vi "Example 3 trig in_out.vi"() -> ()   [LabVIEW 2015]
uses:
  <vilib>/Platform/TimedLoop/XDataNode/timing_clust.ctl
  <vilib>/Platform/TimedLoop/XDataNode/nitl_modes.ctl
  <vilib>/Platform/TimedLoop/XDataNode/wakeup.ctl
  <vilib>/Platform/TimedLoop/XDataNode/XDataNode.xnode
  <vilib>/Platform/TimedLoop/XDataNode/XDNodeRunTimeDep.lvlib
panel:
  out "read 7":dbl
  out "read 6":dbl
  in  "Trigger Out Mode S":u16(ring)=2 items=["OFF", "TRIG", "FSTR"]
  in  "Trigger Out Mode M":u16(ring)=2 items=["OFF", "TRIG", "FSTR"]
  out "resulting string":string="loop -1 from 1"
  out "Counter":dbl=1.0
  in  "Trigger in Delay M(s)":dbl=1.0
  out "full master program time[s]":dbl=4.0
  in  "stop":bool
  in  "Language Selector":i16(ring)=1 items=["GEN", "SCPI"]
  in  "Baud Rate":i32(ring)=6 items=["1200", "2400", "4800", "9600", "19200", "38400", "57600", "115200"]
  in  "Address":i16=6
  out "Read Set Voltage":dbl=5.0
  in  "dt":dbl=0.02 step=0.001 format="%#4_6g"
  in  "time screen\n [SEC]":i16(knob)=10 scale=0.0..60.0
  in  "Trigger in Delay S(s)":dbl=1.0
  out "Waveform Graph":dynamicdata(graph)=[{"t0"=timestamp(0 s since 1904-01-01), "dt"=0.02, "Y"=[-1.0, -1.0, -1.0, -1.0, -1.0, -1.0, -1.0, -1.0, -1.0, -1.0, -1.0, -1.0, -1.0, -1.0, -1.0, -1.0, -1.0, -1.0, -1.0, -1.0, -1.0, -1.0, -1.0, -1.0, -1.0, -1.0, -1.0, -1.0, -1.0, -1.0, -1.0, -1.0, -1.0, -1.0, -1.0, -1.0, -1.0, -1.0, -1.0, -1.0, -1.0, -1.0, -1.0, -1.0, -1.0, -1.0, -1.0, -1.0, -1.0, -1.0, -1.0, -1.0, -1.0, -1.0, -1.0, -1.0, -1.0, -1.0, -1.0, -1.0, -1.0, -1.0, -1.0, -1.0, -1.0, -1.0, -1.0, -1.0, -1.0, -1.0, -1.0, -1.0, -1.0, -1.0, -1.0, -1.0, -1.0, -1.0, -1.0, -1.0, -1.0, -1.0, -1.0, -1.0, -1.0, -1.0, -1.0, -1.0, -1.0, -1.0, -1.0, -1.0, -1.0, -1.0, -1.0, -1.0, -1.0, -1.0, -1.0, -1.0, -1.0, -1.0, -1.0, -1.0, -1.0, -1.0, -1.0, -1.0, -1.0, -1.0, -1.0, -1.0, -1.0, -1.0, -1.0, -1.0, -1.0, -1.0, -1.0, -1.0, -1.0, -1.0, -1.0, -1.0, -1.0, -1.0, -1.0, -1.0, -1.0, -1.0, -1.0, -1.0, -1.0, -1.0, -1.0, -1.0, -1.0, -1.0, -1.0, -1.0, -1.0, -1.0, -1.0, -1.0, -1.0, -1.0, -1.0, -1.0, -1.0, -1.0, -1.0, -1.0, -1.0, -1.0, -1.0, -1.0, -1.0, -1.0, -1.0, -1.0, -1.0, -1.0, -1.0, -1.0, -1.0, -1.0, -1.0, -1.0, -1.0, -1.0, -1.0, -1.0, -1.0, -1.0, -1.0, -1.0, -1.0, -1.0, -1.0, -1.0, -1.0, -1.0, -1.0, -1.0, -1.0, -1.0, -1.0, -1.0, -1.0, -1.0, -1.0, -1.0, -1.0, -1.0, -1.0, -1.0, -1.0, -1.0, -1.0, -1.0, -1.0, -1.0, -1.0, -1.0, -1.0, -1.0, -1.0, -1.0, -1.0, -1.0, -1.0, -1.0, -1.0, -1.0, -1.0, -1.0, -1.0, -1.0, -1.0, -1.0, -1.0, -1.0, -1.0, -1.0, -1.0, -1.0, -1.0, -1.0, -1.0, -1.0, -1.0, -1.0, -1.0, -1.0, -1.0, -1.0, -1.0, -1.0, -1.0, -1.0, -1.0, -1.0, -1.0, -1.0, -1.0, -1.0, -1.0, -1.0, -1.0, -1.0, -1.0, -1.0, -1.0, -1.0, -1.0, -1.0, -1.0, -1.0, -1.0, -1.0, -1.0, -1.0, -1.0, -1.0, -1.0, -1.0, -1.0, -1.0, -1.0, -1.0, -1.0, -1.0, -1.0, -1.0, -1.0, -1.0, -1.0, -1.0, -1.0, -1.0, -1.0, -1.0, -1.0, -1.0, -1.0, -1.0, -1.0, -1.0, -1.0, -1.0, -1.0, -1.0, -1.0, -1.0, -1.0, -1.0, -1.0, -1.0, -1.0, -1.0, -1.0, -1.0, -1.0, -1.0, -1.0, -1.0, -1.0, -1.0, -1.0, -1.0, -1.0, -1.0, -1.0, -1.0, -1.0, -1.0, -1.0, -1.0, -1.0, -1.0, -1.0, -1.0, -1.0, -1.0, -1.0, -1.0, -1.0, -1.0, -1.0, -1.0, -1.0, -1.0, -1.0, -1.0, -1.0, -1.0, -1.0, -1.0, -1.0, -1.0, -1.0, -1.0, -1.0, -1.0, -1.0, -1.0, -1.0, -1.0, -1.0, -1.0, -1.0, -1.0, -1.0, -1.0, -1.0, -1.0, -1.0, -1.0, -1.0, -1.0, -1.0, -1.0, -1.0, -1.0, -1.0, -1.0, -1.0, -1.0, -1.0, -1.0, -1.0, -1.0, -1.0, -1.0, -1.0, -1.0, -1.0, -1.0, -1.0, -1.0, -1.0, -1.0, -1.0, -1.0, -1.0, -1.0, -1.0, -1.0, -1.0, -1.0, -1.0, -1.0, -1.0, -1.0, -1.0, -1.0, -1.0, -1.0, -1.0, -1.0, -1.0, -1.0, -1.0, -1.0, -1.0, -1.0, -1.0, -1.0, -1.0, -1.0, -1.0, -1.0, -1.0, -1.0, -1.0, -1.0, -1.0, -1.0, -1.0, -1.0, -1.0, -1.0, -1.0, -1.0, -1.0, -1.0, -1.0, -1.0, -1.0, -1.0, -1.0, -1.0, -1.0, -1.0, -1.0, -1.0, -1.0, -1.0, -1.0, -1.0, -1.0, -1.0, -1.0, -1.0, -1.0, -1.0, -1.0, -1.0, -1.0, -1.0, -1.0, -1.0, -1.0, -1.0, -1.0, -1.0, -1.0, -1.0, -1.0, -1.0, -1.0, -1.0, -1.0, -1.0, -1.0, -1.0, -1.0, -1.0, -1.0, -1.0, -1.0, -1.0, -1.0, -1.0, -1.0, -1.0, -1.0, -1.0, -1.0, -1.0, -1.0, -1.0, -1.0, -1.0, -1.0, -1.0, -1.0, -1.0, -1.0, -1.0, -1.0, -1.0, -1.0, -1.0, -1.0, -1.0, -1.0, -1.0, -1.0, -1.0]}, {"t0"=timestamp(0 s since 1904-01-01), "dt"=0.02, "Y"=[0.0, 0.0, 0.0, 0.0, 0.0, 0.0, 0.0, 0.0, 0.0, 0.0, 0.0, 0.0, 0.0, 0.0, 0.0, 0.0, 0.0, 0.0, 0.0, 0.0, 0.0, 0.0, 0.0, 0.0, 0.0, 0.0, 0.0, 0.0, 0.0, 0.0, 0.0, 0.0, 0.0, 0.0, 0.0, 0.0, 0.0, 0.0, 0.0, 0.0, 0.0, 0.0, 0.0, 0.0, 0.0, 0.0, 0.0, 0.0, 0.0, 0.0, 0.0, 0.0, 0.0, 0.0, 0.0, 0.0, 0.0, 0.0, 0.0, 0.0, 0.0, 0.0, 0.0, 0.0, 0.0, 0.0, 0.0, 0.0, 0.0, 0.809, 0.809, 1.598, 1.598, 2.408, 2.408, 3.207, 3.207, 4.006, 4.006, 4.805, 4.805, 5.594, 5.594, 6.394, 6.394, 7.203, 7.203, 8.002, 8.002, 8.801, 8.801, 9.6, 9.6, 10.0, 10.0, 10.0, 10.0, 10.0, 10.0, 10.0, 10.0, 10.0, 10.0, 10.0, 10.0, 10.0, 10.0, 10.0, 10.0, 10.0, 10.0, 10.0, 10.0, 10.0, 10.0, 10.0, 10.0, 10.0, 10.0, 10.0, 10.0, 10.0, 10.0, 10.0, 10.0, 10.0, 10.0, 10.0, 10.0, 10.0, 10.0, 10.0, 10.0, 10.0, 10.0, 10.0, 10.0, 10.0, 10.0, 10.0, 10.0, 10.0, 10.0, 9.84, 9.84, 9.52, 9.52, 9.197, 9.197, 8.877, 8.877, 8.557, 8.557, 8.246, 8.246, 7.926, 7.926, 7.602, 7.602, 7.279, 7.279, 6.959, 6.959, 6.639, 6.639, 6.324, 6.324, 6.004, 6.004, 6.0, 6.0, 6.0, 6.0, 6.0, 6.0, 6.0, 6.0, 6.0, 6.0, 6.0, 6.0, 6.0, 6.0, 6.0, 6.0, 6.0, 6.0, 6.0, 6.0, 6.0, 6.0, 6.0, 6.0, 6.0, 6.0, 6.0, 6.0, 6.0, 6.0, 6.0, 6.0, 6.0, 6.0, 6.0, 6.0, 6.0, 6.0, 6.0, 6.0, 6.0, 6.0, 6.0, 6.0, 6.0, 6.0, 6.0, 6.0, 6.0, 6.0, 6.162, 6.162, 6.319, 6.319, 6.481, 6.481, 6.641, 6.641, 6.803, 6.803, 6.957, 6.957, 7.119, 7.119, 7.28, 7.28, 7.44, 7.44, 7.6, 7.6, 7.76, 7.76, 7.922, 7.922, 8.0, 8.0, 8.0, 8.0, 8.0, 8.0, 8.0, 8.0, 8.0, 8.0, 8.0, 8.0, 8.0, 8.0, 8.0, 8.0, 8.0, 8.0, 8.0, 8.0, 8.0, 8.0, 8.0, 8.0, 8.0, 8.0, 8.0, 8.0, 8.0, 8.0, 8.0, 8.0, 8.0, 8.0, 8.0, 8.0, 8.0, 8.0, 8.0, 8.0, 8.0, 8.0, 8.0, 8.0, 8.0, 8.0, 8.0, 8.0]}, {"t0"=timestamp(0 s since 1904-01-01), "dt"=0.02, "Y"=[0.0, 0.0, 0.0, 0.0, 0.0, 0.0, 0.0, 0.0, 0.0, 0.0, 0.0, 0.0, 0.0, 0.0, 0.0, 0.0, 0.0, 0.0, 0.195, 0.195, 0.594, 0.594, 0.999, 0.999, 1.399, 1.399, 1.798, 1.798, 2.203, 2.203, 2.597, 2.597, 2.992, 2.992, 3.396, 3.396, 3.796, 3.796, 4.191, 4.191, 4.59, 4.59, 4.99, 4.99, 5.0, 5.0, 5.0, 5.0, 5.0, 5.0, 5.0, 5.0, 5.0, 5.0, 5.0, 5.0, 5.0, 5.0, 5.0, 5.0, 5.0, 5.0, 5.0, 5.0, 5.0, 5.0, 5.0, 5.0, 5.0, 5.0, 5.0, 5.0, 5.0, 5.0, 5.0, 5.0, 5.0, 5.0, 5.0, 5.0, 5.0, 5.0, 5.0, 5.0, 5.0, 5.0, 5.0, 5.0, 5.0, 5.0, 5.0, 5.0, 5.0, 5.0, 4.84, 4.84, 4.68, 4.68, 4.518, 4.518, 4.358, 4.358, 4.198, 4.198, 4.041, 4.041, 3.881, 3.881, 3.719, 3.719, 3.559, 3.559, 3.399, 3.399, 3.241, 3.241, 3.08, 3.08, 3.0, 3.0, 3.0, 3.0, 3.0, 3.0, 3.0, 3.0, 3.0, 3.0, 3.0, 3.0, 3.0, 3.0, 3.0, 3.0, 3.0, 3.0, 3.0, 3.0, 3.0, 3.0, 3.0, 3.0, 3.0, 3.0, 3.0, 3.0, 3.0, 3.0, 3.0, 3.0, 3.0, 3.0, 3.0, 3.0, 3.0, 3.0, 3.0, 3.0, 3.0, 3.0, 3.0, 3.0, 3.0, 3.0, 3.0, 3.0, 3.0, 3.0, 3.04, 3.04, 3.12, 3.12, 3.201, 3.201, 3.28, 3.28, 3.36, 3.36, 3.438, 3.438, 3.519, 3.519, 3.6, 3.6, 3.68, 3.68, 3.76, 3.76, 3.84, 3.84, 3.92, 3.92, 3.999, 3.999, 4.0, 4.0, 4.0, 4.0, 4.0, 4.0, 4.0, 4.0, 4.0, 4.0, 4.0, 4.0, 4.0, 4.0, 4.0, 4.0, 4.0, 4.0, 4.0, 4.0, 4.0, 4.0, 4.0, 4.0, 4.0, 4.0, 4.0, 4.0, 4.0, 4.0, 4.0, 4.0, 4.0, 4.0, 4.0, 4.0, 4.0, 4.0, 4.0, 4.0, 4.0, 4.0, 4.0, 4.0, 4.0, 4.0, 4.0, 4.0, 4.0, 4.0, 4.079, 4.079, 4.159, 4.159, 4.24, 4.24, 4.321, 4.321, 4.401, 4.401, 4.479, 4.479, 4.559, 4.559, 4.64, 4.64, 4.72, 4.72, 4.8, 4.8, 4.88, 4.88, 4.961, 4.961, 5.0, 5.0, 5.0, 5.0, 5.0, 5.0, 5.0, 5.0, 5.0, 5.0, 5.0, 5.0, 5.0, 5.0, 5.0, 5.0, 5.0, 5.0, 5.0, 5.0, 5.0, 5.0, 5.0]}]
  in  "Boolean":bool
  in  "S DATA":T1={"Value string"="10,6,8", "Time string"="1,1,1", "step"=0, "Counter"=1.0} {"Counter" min=1.0 max=65534.0 step=1.0; "step" items=["ONCE", "AUTO"]}
  in  "S MODE":T2={"Progr Mode"=3, "Mode"=0, "init:cont"=1} {"init:cont" items=["0", "1"]; "Mode" items=["VOLTAGE", "CURRENT"]; "Progr Mode" items=["NONE", "FIX", "LIST", "WAVE"]}
  in  "M DATA":T1={"Value string"="5,3,4", "Time string"="1,1,1", "step"=0, "Counter"=1.0} {"Counter" min=1.0 max=65534.0 step=1.0; "step" items=["ONCE", "AUTO"]}
  in  "M MODE":T2={"Progr Mode"=3, "Mode"=0, "init:cont"=1} {"init:cont" items=["0", "1"]; "Mode" items=["VOLTAGE", "CURRENT"]; "Progr Mode" items=["NONE", "FIX", "LIST", "WAVE"]}
  in  "VISA":refnum<visa-resource-name>="COM10"
  # "Application for two power supplies connected\ndaisy chain with Tr_IN and TR_Out"
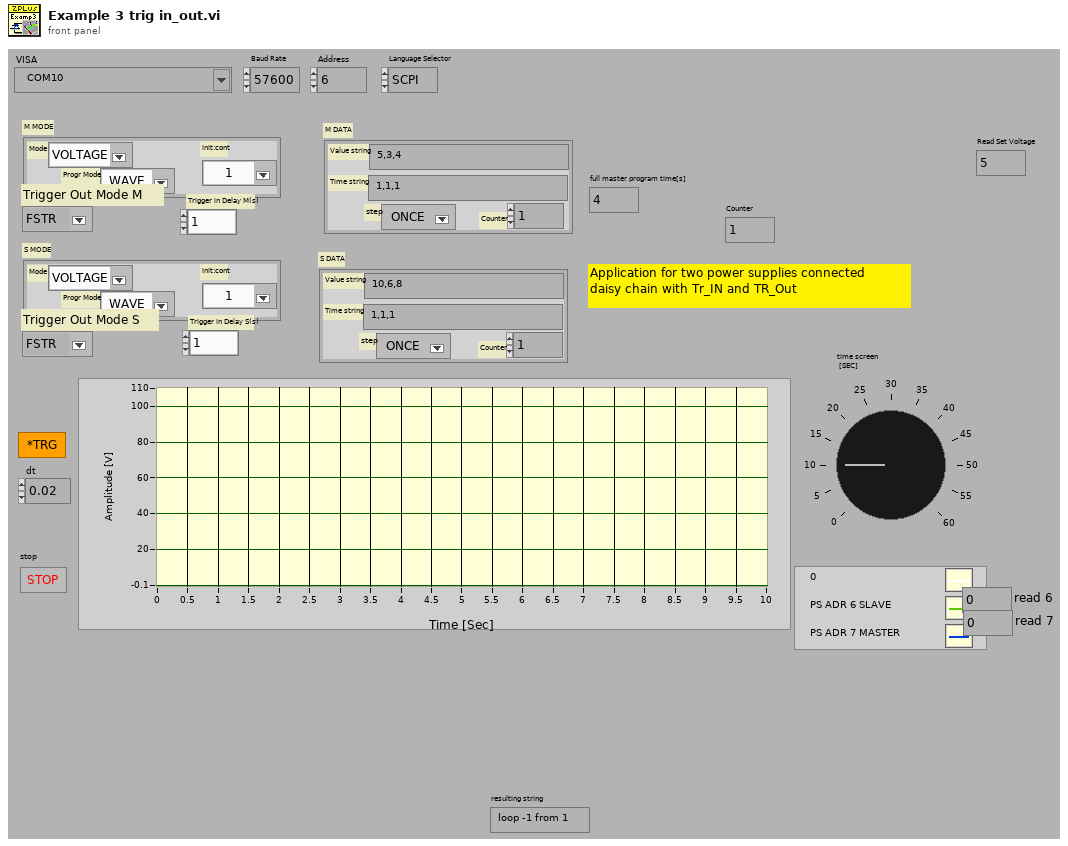
[diagram p1: front panel]
types:
  T1 = cluster{"Value string":string, "Time string":string, "step":u16, "Counter":dbl}
  T2 = cluster{"Progr Mode":u16, "Mode":u16, "init:cont":u16}
  T3 = typedef "XDNodeRunTimeDep.lvlib/timing_clust.ctl" = cluster{"Expected End [f-1]":u64, "Actual End [f-1]":u64, "Finished Late? [f-1]":bool, "Expected End [i-1]":u64, "Actual End [i-1]":u64, "Finished Late? [i-1]":bool, "Expected Start [i]":u64, "Actual Start [i]":u64, "Expected Start [f]":u64, "Actual Start [f]":u64, "Source Name":string, "Structure Name":string, "Period":i64, "Deadline":i64, "Offset":i64, "Start":i64, "Priority":i32, "Timeout":i32, "Mode":T4, "Wakeup Reason":T5, "Error":errorcluster, "Source Type":string, "Secondary Source Type":string, "Global End Time":u64, "Global Start Time":u64, "Frame Duration":u64, "Iteration Duration":u64, "Assigned CPU":i32, "I/O Scan Engine Mode":u32}
  T4 = typedef "XDNodeRunTimeDep.lvlib/nitl_modes.ctl" = enum32{"No Change", "Process missed periods, maintain original phase", "Discard missed periods, maintain original phase", "Process missed periods, ignore original phase", "Discard missed periods, ignore original phase"}
  T5 = typedef "XDNodeRunTimeDep.lvlib/wakeup.ctl" = enum32{"Normal", "Aborted", "Asynchronous wakeup", "Timing source error", "Timed loop error", "Timeout"}
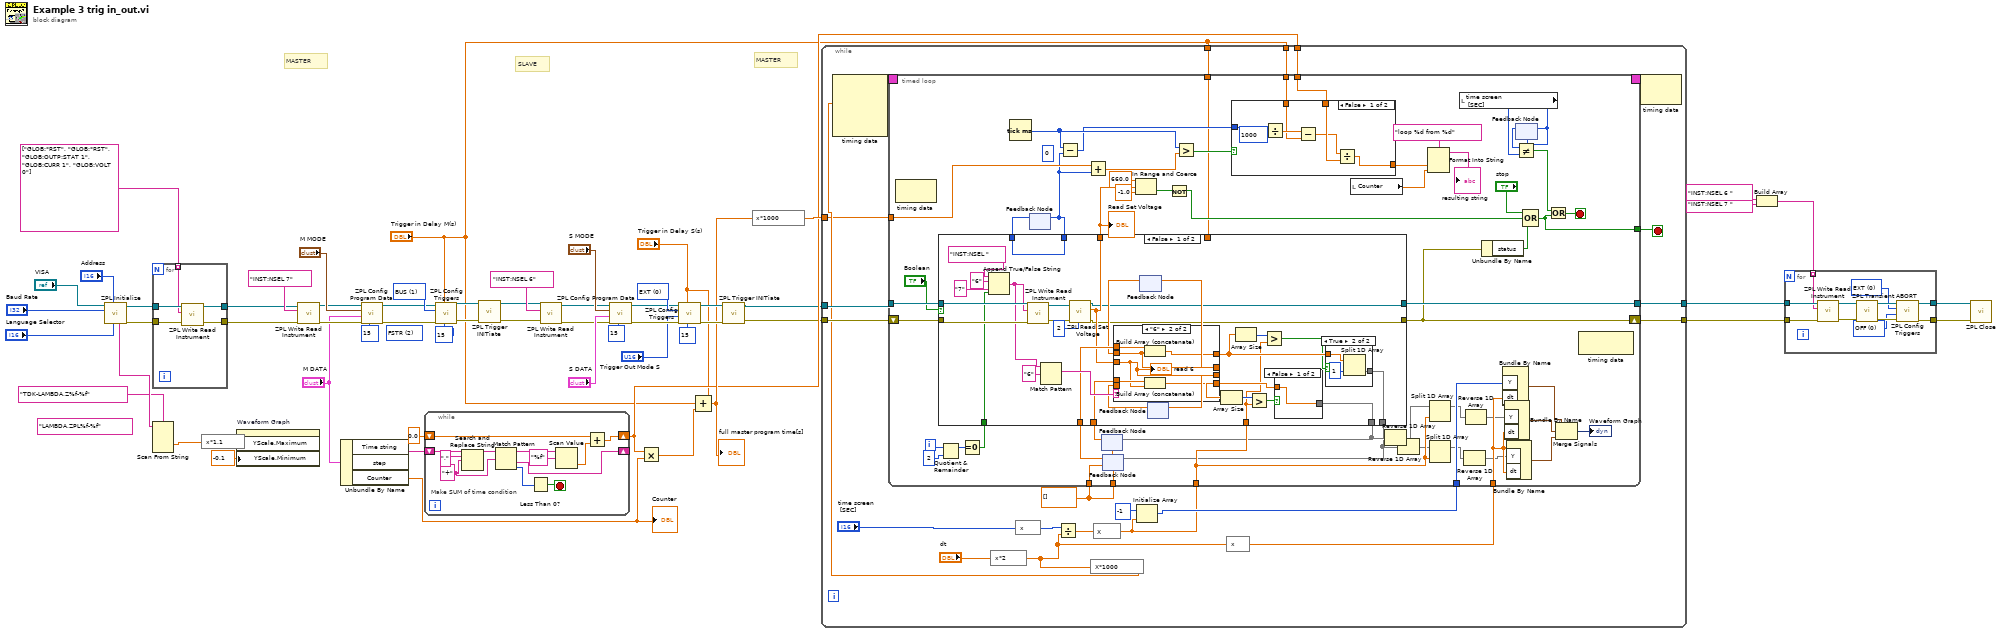
[diagram p0: block diagram]
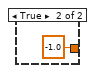
[diagram p2: hidden frame]
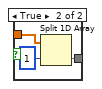
[diagram p4: hidden frame]
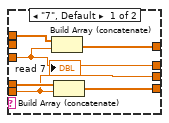
[diagram p5: hidden frame]
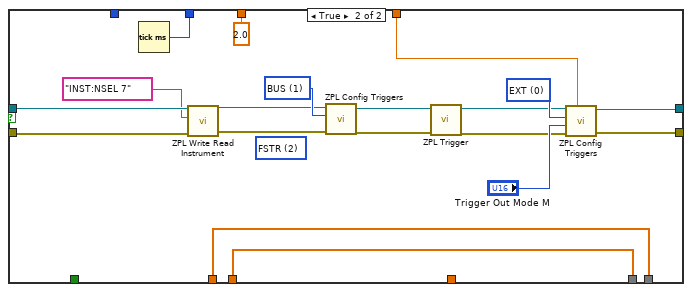
[diagram p6: hidden frame]
diagram:
  (unwired) "LAMBDA,ZPL%f-%f" ("format string")
  (unwired) u16 2 items=["OFF", "TRIG", "FSTR"] ("Trigger Out Mode")
  w50 = u16 0 items=["EXT", "BUS"] ("Trigger in  Source")
  w54 = u16 1 items=["EXT", "BUS"] ("Trigger in  Source")
  # "MASTER"
  # "SLAVE"
  # "MASTER"
  n1 = call "ZPL Initialize.vi"("Language Selector"="Language Selector", "Address"="Address", "Baud Rate"="Baud Rate", "VISA"="VISA") -> ("error out"=w34:errorcluster, "VISA  out"=w33:refnum<visa-resource-name>, "ID responce"=w25:string)  [unwired: 4 in, 1 out]
  n2 = Scan From String(format string="TDK-LAMBDA,Z%f-%f", input string=w25) -> (output 1=w24:dbl)  [unwired: 5 in, 3 out]
  n3 = for {
    tunnel: w34 -> [w64]
    tunnel: w33 -> [w63]
    tunnel: [w62] -> w32
    tunnel: [w61] -> w31
    tunnel: string[] ["GLOB:*RST", "GLOB:*RST", "GLOB:OUTP:STAT 1", "GLOB:CURR 1", "GLOB:VOLT 0"] -> [w60] mode=indexing
    n4 = call "ZPL Write Read Instrument.vi"("error in"=w64, "Write Command/Query SCPI"=w60, "VISA"=w63) -> ("error out"=w61:errorcluster, "VISA  out"=w62:refnum<visa-resource-name>)  [unwired: 6 in, 1 out]
  }
  n5 = expression code="x*1.1"(w24) -> (w23:dbl)
  n6 = property on="Waveform Graph" class="WFGraph (strict)"("YScale.Maximum"=w23, "YScale.Minimum"=-0.1 ("Y Scale.Range:Minimum")) -> ()  [unwired: 2 in, 2 out]
  n7 = call "ZPL Write Read Instrument.vi"("error in"=w31, "Write Command/Query SCPI"="INST:NSEL 7", "VISA"=w32) -> ("error out"=w29:errorcluster, "VISA  out"=w30:refnum<visa-resource-name>)  [unwired: 6 in, 1 out]
  n8 = Unbundle By Name("M DATA") -> ("Time string"=w20:string, "Counter"=w15:dbl)  [unwired: 1 out]
  "Counter" <- w15
  n9 = call "ZPL Config Program Data.vi"("Settle (1 mS)"=u32 15, "error"=w29, "DATA"="M DATA", "MODE"="M MODE", "VISA"=w30) -> ("error out"=w52:errorcluster, "VISA out"=w53:refnum<visa-resource-name>)  [unwired: 4 in, 1 out]
  n10 = while {
    shift-right: [w74] -> _
    shift-left: w20 -> [w73]
    shift-right: [w67] -> w14
    shift-left: 0.0 -> [w66]
    stop <- w71 stop-if-true
    w65 = "+" ("search string")
    # "Make SUM of time condition"
    n11 = Search and Replace String(input string=w73, search string=",", replace string=w65) -> (result string=w75:string)  [unwired: 5 in, 3 out]
    n12 = Match Pattern(string=w75, regular expression=w65) -> (before substring=w69:string, after substring=w74:string, offset past match=w72:i32)  [unwired: 1 in, 1 out]
    n13 = Less Than 0?(x=w72) -> (x < 0?=w71:bool)
    n14 = Scan Value(string=w69, format string="%f") -> (value=w68:dbl)  [unwired: 1 in, 1 out]
    n15 = Add(x=w66, y=w68) -> (x+y=w67:dbl)
  }
  n16 = call "ZPL Config Triggers.vi"("Settle (1 mS)"=u32 15, "Trigger in Delay"="Trigger in Delay M(s)", "error"=w52, "Trigger in  Source"=w54, "VISA"=w53) -> ("error out"=w43:errorcluster, "VISA out"=w44:refnum<visa-resource-name>)  [unwired: 4 in, 1 out]
  n17 = call "ZPL Trigger INITiate.vi"("error"=w43, "VISA"=w44) -> ("error out"=w38:errorcluster, "VISA out"=w42:refnum<visa-resource-name>)  [unwired: 8 in]
  n18 = call "ZPL Write Read Instrument.vi"("error in"=w38, "Write Command/Query SCPI"="INST:NSEL 6", "VISA"=w42) -> ("error out"=w27:errorcluster, "VISA  out"=w28:refnum<visa-resource-name>)  [unwired: 6 in, 1 out]
  n19 = call "ZPL Config Program Data.vi"("Settle (1 mS)"=u32 15, "error"=w27, "DATA"="S DATA", "MODE"="S MODE", "VISA"=w28) -> ("error out"=w48:errorcluster, "VISA out"=w49:refnum<visa-resource-name>)  [unwired: 4 in, 1 out]
  n20 = Multiply(x=w14, y=w15) -> (x*y=w18:dbl)
  n21 = call "ZPL Config Triggers.vi"("Settle (1 mS)"=u32 15, "Trigger in Delay"="Trigger in Delay S(s)", "error"=w48, "Trigger Out Mode"="Trigger Out Mode S", "Trigger in  Source"=w50, "VISA"=w49) -> ("error out"=w40:errorcluster, "VISA out"=w41:refnum<visa-resource-name>)  [unwired: 3 in, 1 out]
  n22 = Compound Arithmetic op=ADD("Trigger in Delay S(s)", "Trigger in Delay M(s)", w18) -> (w17:dbl)
  "full master program time[s]" <- w17
  n23 = call "ZPL Trigger INITiate.vi"("error"=w40, "VISA"=w41) -> ("error out"=w3:errorcluster, "VISA out"=w4:refnum<visa-resource-name>)  [unwired: 8 in]
  n24 = expression code="x*1000"(w17) -> (w19:dbl)
  n25 = while {
    tunnel: [w96] -> w11
    tunnel: [w95] -> w12
    tunnel: w4 -> [w94]
    tunnel: w3 -> [w93]
    tunnel: w19 -> [w81]
    tunnel: w14 -> [w80]
    tunnel: "Trigger in Delay M(s)" -> [w79]
    tunnel: "Trigger in Delay M(s)" -> [w77]
    stop <- w82 stop-if-true
    w91 = dbl[] []
    n26 = expression code="x*2"("dt") -> (w78:dbl)
    n27 = expression code="x"("time screen\n [SEC]") -> (w83:i16)
    n28 = Divide(x=w83, y=w78) -> (x/y=w89:dbl)
    n29 = expression code="X*1000"(w78) -> (w87:dbl)
    n30 = node-c288(w87) -> (w98:T3)  [unwired: 3 in]
    n31 = expression code="X"(w89) -> (w86:dbl)
    n32 = Initialize Array(-1 ("Read Set Voltage"), w86) -> (w90:i32[])
    n33 = expression code="x"(w78) -> (w85:dbl)
    n34 = timed-loop {
      tunnel: w94 -> [w152]
      tunnel: [w136] -> w96
      tunnel: w91 -> [w140]
      tunnel: w91 -> [w139]
      tunnel: w90 -> [w138]
      tunnel: w85 -> [w137]
      tunnel: w86 -> [w108]
      timing: w98 -> [_]
      timing-out: [_] -> w97
      shift-right: [w135] -> w95
      shift-left: w93 -> [w151]
      tunnel: [w125] -> w82
      tunnel: w81 -> [w120]
      tunnel: w80 -> [w114]
      tunnel: w79 -> [w113]
      tunnel: w77 -> [w99]
      i -> [w149]
      stop <- w126 stop-if-true
      (unwired) u32 0 ("y")
      n35 = node-c288() -> ()  [unwired: 1 in, 1 out]
      n36 = Quotient & Remainder(x=w149, y=2) -> (x-y*floor(x/y)=w147:i32)  [unwired: 1 out]
      n37 = Equal To 0?(x=w147) -> (x = 0?=w146:bool)
      n38 = Tick Count (ms)() -> (millisecond timer value=w118:u32)
      n39 = feedback #1() -> (w121:u32)  [unwired: 1 in]
      n40 = feedback #2(w139) -> (w145:dbl[])
      n41 = feedback #3(w140) -> (w144:dbl[])
      n42 = case shown="False" "Boolean" {
        tunnel: w152 -> [w193 w217]
        tunnel: w151 -> [w192 w216]
        tunnel: [w165 w223] -> w136
        tunnel: [w164 w222] -> w135
        tunnel: w146 -> [w189 _]
        tunnel: [w178 w232] -> w107
        tunnel: w145 -> [w182 w232]
        tunnel: [w176 w231] -> w106
        tunnel: w144 -> [w181 w231]
        tunnel: w108 -> [w172 _]
        tunnel: [w167 2.0 ("Read Set Voltage")] -> w133
        tunnel: [w166 w229] -> w117
        tunnel: w121 -> [w166 _]
        tunnel: w99 -> [_ w214]
        frame False {
          n43 = Append True/False String(1:w189, 2:"7" ("false string"), 3:"6" ("true string"), 4:"INST:NSEL " ("Write Command/Query SCPI")) -> (0:w183:string)
          n44 = call "ZPL Write Read Instrument.vi"("error in"=w192, "Write Command/Query SCPI"=w183, "VISA"=w193) -> ("error out"=w190:errorcluster, "VISA  out"=w191:refnum<visa-resource-name>)  [unwired: 6 in, 1 out]
          n45 = Match Pattern(string=w183, regular expression="6") -> (match substring=w185:string)  [unwired: 1 in, 3 out]
          n46 = call "ZPL Read Set Voltage.vi"("Settle (1 mS)"=u32 2, "error"=w190, "VISA"=w191) -> ("error out"=w164:errorcluster, "Read Set Voltage"=w167:dbl, "VISA out"=w165:refnum<visa-resource-name>)  [unwired: 6 in]
          n47 = feedback #4() -> (w171:dbl)  [unwired: 1 in]
          n48 = feedback #5() -> (w170:dbl)  [unwired: 1 in]
          n49 = case shown="\"6\"" w185 {
            tunnel: w167 -> [w203 w209]
            tunnel: [w204 w213] -> w179
            tunnel: [w207 w211] -> w174
            tunnel: w182 -> [w205 w212]
            tunnel: w181 -> [w206 w210]
            tunnel: [w203 w208] -> w169
            tunnel: w171 -> [_ w208]
            tunnel: w170 -> [w202 _]
            tunnel: [w202 w209] -> w168
            frame "7", Default {
              n50 = Build Array (concatenate)(w206, w203) -> (w207:dbl[])
              n51 = Build Array (concatenate)(w205, w202) -> (w204:dbl[])
              "read 7" <- w203
            }
            frame "6" {
              n52 = Build Array (concatenate)(w210, w208) -> (w211:dbl[])
              n53 = Build Array (concatenate)(w212, w209) -> (w213:dbl[])
              "read 6" <- w209
            }
          }
          n54 = feedback-in #4(w169) -> ()
          n55 = feedback-in #5(w168) -> ()
          n56 = Array Size(array=w179) -> (size(s)=w180:i32)
          n57 = Array Size(array=w174) -> (size(s)=w175:i32)
          n58 = Greater?(x=w180, y=w172) -> (0:w177:bool)
          n59 = Greater?(x=w175, y=w172) -> (0:w173:bool)
          n60 = case shown="False" w177 {
            tunnel: w179 -> [w198 w200]
            tunnel: [w198 w199] -> w178
            frame False {
            }
            frame True {
              n61 = Split 1D Array(array=w200, index=1) -> (second subarray=w199:dbl[])  [unwired: 1 out]
            }
          }
          n62 = case shown="True" w173 {
            tunnel: w174 -> [w194 w196]
            tunnel: [w194 w195] -> w176
            frame False {
            }
            frame True {
              n63 = Split 1D Array(array=w196, index=1) -> (second subarray=w195:dbl[])  [unwired: 1 out]
            }
          }
        }
        frame True {
          w225 = u16 0 items=["EXT", "BUS"] ("Trigger in  Source")
          (unwired) u16 2 items=["OFF", "TRIG", "FSTR"] ("Trigger Out Mode")
          w228 = u16 1 items=["EXT", "BUS"] ("Trigger in  Source")
          n64 = Tick Count (ms)() -> (millisecond timer value=w229:u32)
          n65 = call "ZPL Write Read Instrument.vi"("error in"=w216, "Write Command/Query SCPI"="INST:NSEL 7", "VISA"=w217) -> ("error out"=w218:errorcluster, "VISA  out"=w219:refnum<visa-resource-name>)  [unwired: 6 in, 1 out]
          n66 = call "ZPL Config Triggers.vi"("error"=w218, "Trigger in  Source"=w228, "VISA"=w219) -> ("error out"=w226:errorcluster, "VISA out"=w227:refnum<visa-resource-name>)  [unwired: 6 in, 1 out]
          n67 = call "ZPL Trigger.vi"("error"=w226, "VISA"=w227) -> ("error out"=w221:errorcluster, "VISA out"=w220:refnum<visa-resource-name>)  [unwired: 8 in]
          n68 = call "ZPL Config Triggers.vi"("Trigger in Delay"=w214, "error"=w221, "Trigger Out Mode"="Trigger Out Mode M", "Trigger in  Source"=w225, "VISA"=w220) -> ("error out"=w222:errorcluster, "VISA out"=w223:refnum<visa-resource-name>)  [unwired: 4 in, 1 out]
        }
      }
      "Read Set Voltage" <- w133
      n69 = feedback-in #1(w117) -> ()
      n70 = Subtract(x=w118, y=w117) -> (x-y=w115:u32)
      n71 = Add(x=w120, y=w117) -> (x+y=w119:dbl)
      n72 = feedback-in #2(w107) -> ()
      n73 = feedback-in #3(w106) -> ()
      n74 = In Range and Coerce(upper limit=660.0, x=w133, lower limit=-1.0) -> (In Range?=w130:bool)  [unwired: 1 out]
      n75 = Not(x=w130) -> (.not. x?=w128:bool)
      n76 = Greater?(x=w118, y=w119) -> (0:w116:bool)
      n77 = case shown="False" w116 {
        tunnel: w115 -> [w159 _]
        tunnel: w114 -> [w157 _]
        tunnel: w113 -> [w154 _]
        tunnel: [w153 -1.0] -> w111
        frame False {
          n78 = Divide(x=w159, y=u32 1000) -> (x/y=w156:dbl)
          n79 = Subtract(x=w156, y=w154) -> (x-y=w155:dbl)
          n80 = Divide(x=w155, y=w157) -> (x/y=w153:dbl)
        }
        frame True {
        }
      }
      n81 = local read "Counter"() -> (w110:dbl)
      n82 = Reverse 1D Array(array=w107) -> (reversed array=w105:dbl[])
      n83 = Reverse 1D Array(array=w106) -> (reversed array=w104:dbl[])
      n84 = Format Into String(format string="loop %d from %d", w111, w110) -> (resulting string=→"resulting string":string)  [unwired: 2 in, 1 out]
      n85 = Split 1D Array(array=w105, index=w108) -> (first subarray=w101:dbl[])  [unwired: 1 out]
      n86 = Split 1D Array(array=w104, index=w108) -> (first subarray=w100:dbl[])  [unwired: 1 out]
      n87 = local read "time screen\n [SEC]"() -> (w122:i16)
      n88 = Reverse 1D Array(array=w100) -> (reversed array=w102:dbl[])
      n89 = Reverse 1D Array(array=w101) -> (reversed array=w103:dbl[])
      n90 = Unbundle By Name(w135) -> ("status"=w129:bool)
      n91 = Bundle By Name("Y"=w138, "dt"=w137) -> (w134:waveform(i32))  [unwired: 1 in]
      n92 = Bundle By Name("Y"=w103, "dt"=w137) -> (w143:waveform(dbl))  [unwired: 1 in]
      n93 = Bundle By Name("Y"=w102, "dt"=w137) -> (w142:waveform(dbl))  [unwired: 1 in]
      n94 = feedback-in #6(w122) -> ()
      n95 = feedback #6(w122) -> (w124:i16)
      n96 = Not Equal?(x=w124, y=w122) -> (x != y?=w123:bool)
      n97 = Compound Arithmetic op=OR("stop", w128, w129) -> (w125:bool)
      n98 = Or(x=w123, y=w125) -> (x .or. y?=w126:bool)
      n99 = Merge Signals(w134, w143, w142) -> (→"Waveform Graph":dynamicdata)
      n100 = node-c288() -> ()  [unwired: 1 in, 1 out]
    }
    n101 = node-c288(w97) -> ()  [unwired: 1 out]
  }
  n102 = Build Array("INST:NSEL 6 " ("Write Command/Query SCPI"), "INST:NSEL 7 " ("Write Command/Query SCPI")) -> (w6:string[])
  n103 = for {
    tunnel: w12 -> [w247]
    tunnel: w11 -> [w246]
    tunnel: [w240] -> w10
    tunnel: [w239] -> w9
    tunnel: w6 -> [w243] mode=indexing
    w237 = u16 0 items=["EXT", "BUS"] ("Trigger in  Source")
    w238 = u16 0 items=["OFF", "TRIG", "FSTR"] ("Trigger Out Mode")
    n104 = call "ZPL Write Read Instrument.vi"("error in"=w247, "Write Command/Query SCPI"=w243, "VISA"=w246) -> ("error out"=w244:errorcluster, "VISA  out"=w245:refnum<visa-resource-name>)  [unwired: 6 in, 1 out]
    n105 = call "ZPL Transient ABORT.vi"("error"=w244, "VISA"=w245) -> ("error out"=w241:errorcluster, "VISA out"=w242:refnum<visa-resource-name>)  [unwired: 8 in]
    n106 = call "ZPL Config Triggers.vi"("error"=w241, "Trigger Out Mode"=w238, "Trigger in  Source"=w237, "VISA"=w242) -> ("error out"=w239:errorcluster, "VISA out"=w240:refnum<visa-resource-name>)  [unwired: 5 in, 1 out]
  }
  n107 = call "ZPL Close.vi"("error"=w9, "VISA name"=w10) -> ()  [unwired: 7 in, 1 out]
